vi "Get Proj Item Ref from VI Name.vi"(0 "ProjectI tem":refnum<vi>, 5 "VI Name":string, 11 "error in (no error)":errorcluster) -> (4 "VI Project Item Reference":refnum<vi>, 6 "Found":bool, 15 "error out":errorcluster)   [LabVIEW 2020, in "MVA Message Mapper.lvlib"]
uses:
  <vilib>/gpm_packages/@cs/Bus-message-mapper/Source/MVA Message Mapper.lvlib
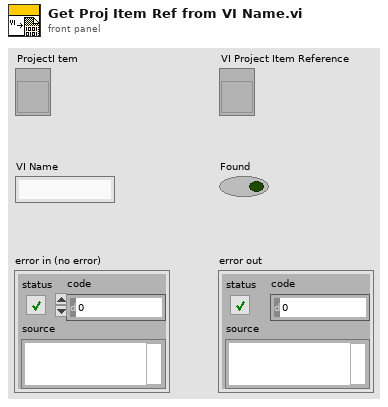
[diagram p1: front panel]
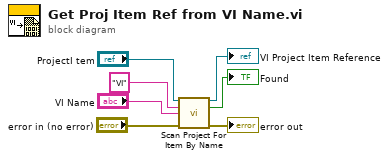
[diagram p0: block diagram]
diagram:
  n1 = call <vilib>:"Scan Project For Item By Name.vi"("ProjectItem in"="ProjectI tem", "Type"="VI", "Item Name"="VI Name", "error in (no error)"="error in (no error)") -> ("ProjectItem out"=→"VI Project Item Reference":refnum<vi>, "Found"=→"Found":bool, "error out"=→"error out":errorcluster)  [unwired: 9 in]
